vi "OpenCLV Manual and Examples.vi"   [LabVIEW 2012]
uses:
  <vilib>/Platform/browser.llb/Open URL in Default Browser (path).vi
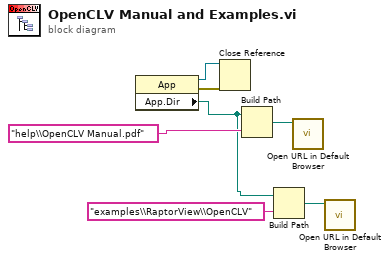
[diagram p0: block diagram]
diagram:
  n1 = property class="App"() -> (reference out=w4:refnum<vi>, error out=w5:errorcluster, "App.Dir"=w1:path)  [unwired: 2 in]
  n2 = Close Reference(reference=w4, error in (no error)=w5) -> ()  [unwired: 1 out]
  n3 = Build Path(base path=w1, name or relative path="help\\OpenCLV Manual.pdf") -> (appended path=w6:path)
  n4 = Build Path(base path=w1, name or relative path="examples\\RaptorView\\OpenCLV") -> (appended path=w2:path)
  n5 = call-poly <vilib>:"Open URL in Default Browser.vi"("path"=w6) -> ()  [unwired: 5 in, 2 out]
  n6 = call-poly <vilib>:"Open URL in Default Browser.vi"("path"=w2) -> ()  [unwired: 5 in, 2 out]
